vi "VI Linearisierung v2.vi"() -> ()   [LabVIEW 2020, in "Linearisierung v2.lvlib"]
uses:
  Linearisierung v2.lvlib
  Gasteiler/Stufen Tabelle.ctl
  Visualisierungs Elemente/Button.ctl
  Parameterkontrolle.ctl
  Visualisierungs Elemente/String - Eingabefeld.ctl
  SpanEinstellungen/SpanInletCluster.ctl
  Seiten/System Einstellungen V2/Konfig Gasflasche.ctl
  Seiten/System Einstellungen V2/Analysatoren.ctl
  Seiten/System Einstellungen V2/Gasflasche Auswahl.ctl
  SpanEinstellungen/Komponentencluster mit Formel.ctl
  SpanEinstellungen/Komponentenauswahl mit Formel.ctl
  SpanEinstellungen/Einheit.ctl
  Seiten/System Einstellungen V2/Traegergas.ctl
  Gasteiler/Gasteiler Stufen.ctl
  GasteilerType.ctl
  Visualisierungs Elemente/Zahlen-Ausgabefeld.ctl
  Gasteiler/Gasteiler Fehler.ctl
  Gasteiler/RS232.ctl
  Eingabetabelle.ctl
  Ausgabetabelle.ctl
  Auswahl Polynom Ordnung.ctl
  LIN Ausgabetabelle.ctl
  Visualisierungs Elemente/String - Ausgabefeld.ctl
  Gasnumber.ctl
  AktivArray.ctl
  AktivButton.ctl
  EPA Ausgabetabelle.ctl
  Visualisierungs Elemente/Pfad-Eingabefeld.ctl
  EPA Optionsfeld.ctl
  Gasteiler/HovaCal/Betriebsdaten.ctl
  Gasteiler/HovaCal/Gase.ctl
  Gasteiler/HovaCal/Vaporizer.ctl
  Gasteiler/HovaCal/Dynamsiche_Werte.ctl
  Polynomkoeffizientenanzeige.ctl
  Gasteiler/HovaCal/AutoLin Hovacal.ctl
  Seiten/CalGas Aufschaltung/Aufschaltung CalGas_ANZEIGE.ctl
  Visualisierungs Elemente/Auswahlfeld.ctl
  Kalibrieroption.ctl
  EPA1065-307/Condition.ctl
  Seiten/System Einstellungen V2/Gasteiler Auswahl.ctl
  Gasteiler/HovaCAL_Interface/Controls/Info Cluster Anzeige.ctl
  Gasteiler/HovaCAL_Interface/Controls/MFC Flow Anzeige.ctl
  Gasteiler/HovaCAL_Interface/Controls/Grenzen Anzeige.ctl
  Gasteiler/HovaCAL_Interface/Controls/Pumpe Modus Anzeige.ctl
  Gasteiler/HovaCAL_Interface/Controls/Pump Dry Mode Anzeige.ctl
  Gasteiler/HovaCAL_Interface/Controls/Pump Control Mode Anzeige.ctl
  Gasteiler/HovaCAL_Interface/Controls/Temp Ausgang Anzeige.ctl
  Gasteiler/HovaCAL_Interface/Controls/Temp Sollwerte Anzeige.ctl
  Gasteiler/HovaCAL_Interface/Controls/Flow Einstellung.ctl
  Gasteiler/HovaCAL_Interface/Controls/Flow Anzeige.ctl
  Gasteiler/HovaCAL_Interface/Controls/Pumpe Status Anzeige.ctl
  Gasteiler/HovaCAL_Interface/Controls/Pump state.ctl
  Gasteiler/HovaCAL_Interface/Controls/Pumpe MassenFluss Anzeige.ctl
  Gasteiler/HovaCAL_Interface/Controls/Pumpen Parameter Anzeige.ctl
  Gasteiler/HovaCAL_Interface/Controls/Reagent Anzeige.ctl
  Gasteiler/HovaCAL_Interface/Controls/Pump Concentration Mode Anzeige.ctl
  Gasteiler/HovaCAL_Interface/Controls/MFC Konfiguration.ctl
  Gasteiler/HovaCAL_Interface/Controls/MFC Einstellungen.ctl
  Gasteiler/HovaCAL_Interface/Controls/MFC Output.ctl
  Gasteiler/HovaCAL_Interface/Controls/Pumpen Output.ctl
  Visualisierungs Elemente/Checkbox(boolsch).ctl
  Seiten/CalGas Aufschaltung/Lin Modus.ctl
  Gasteiler/HovaCAL_Interface/Controls/Pumpen Parameter Anzeige Eingabe.ctl
  EPA 1065/T90 1065-308/Auswahl.ctl
  SpanEinstellungen/Aktion FGV Komponentenreferenz verwalten.ctl
  Seiten/FT-IR/FGV FT-IR Gasliste Aktionen.ctl
  Seiten/System Einstellungen V2/Aktion FGV Gasbottledefinition.ctl
  SpanEinstellungen/Aktion FGV SpanEinstellungen.ctl
  SpanEinstellungen/Aktion FGV Spans abarbeiten.ctl
  SpanEinstellungen/Aktion FGV SPAN Verriegelung.ctl
  Gasteiler/Aktion FGV Gasteilerliste laden.ctl
  SpanEinstellungen/Aktion FGV Post Processing.ctl
  SpanEinstellungen/Aktion FGV SPAN Stufentabellen.ctl
  Gasteiler/HovaCAL_Interface/Kommunikation/Aktion_FGV_HovaCAL_Interface_Kommandos.ctl
  Gasteiler/HovaCAL_Interface/Kommunikation/Aktion_FGV_HovaCAL_Interface_GetData.ctl
  Gasteiler/HovaCAL_Interface/Kommunikation/Aktion_FGV_HovaCAL_Interface_SetData.ctl
  Aktion Lin Daten aufarbeiten.ctl
  Gasteiler/Gasteiler Type.ctl
  Gasteiler/HovaCal/Aktion_FGV_Betriebsdaten.ctl
  LinV2 Registerkarten.ctl
  Seiten/CalGas Aufschaltung/FGV CalGas Aktionen.ctl
  Seiten/FT-IR/Span/Aktion FGV Span.ctl
  Gasteiler/Aktionen FGV Gasteiler Daten.ctl
  Aktion FGV Stoerungen sammeln und auswerten.ctl
  Aktion FGV Rohmesswerte sammeln.ctl
  Gasteiler/HovaCAL_Interface/Kommunikation/Aktion FGV HovaCAL Interface Autolin.ctl
  Aktionen Polynom Daten speichern.ctl
  Gasteiler/Aktion FGV Gasteiler Korrektur.ctl
  Gasteiler/Aktion FGV Daten Abholung uebergebenctl.ctl
  Gasteiler/HovaCAL_Interface/Kommunikation/Aktion_FGV_HovaCAL_Interface_Kommunikation.ctl
  Sprachverwaltung/FGV Aktion Tabelle zerlegen.ctl
  PDF_Interface/PDF Interface Helper/PDFResultPictures.ctl
  Seiten/FT-IR/Aktionen EVID-Codes.ctl
  EPA 1065/Allgemeine VIs/Aktion Wertaenderung Gasliste.ctl
  EPA 1065/Allgemeine VIs/Aktion Test Status.ctl
  Passwortverwaltung/FGV Passwort Aktion.ctl
  Gasteiler/AK-Komm Gasteiler/Aktionen AK Komm.ctl
  Gasteiler/AK-Komm Gasteiler/Alter Gasteiler/Aktionen AK Komm_ALT.ctl
  Gasteiler/Horiba/Aktion Befehl.ctl
  Gasteiler/HovaCAL_Interface/Kommunikation/Aktion_FGV_HovaCAL_Interface_Gasliste.ctl
  Seiten/System Einstellungen V2/Aktion FGV SystemEinstellungenV2.ctl
  Gasteiler/Gasteiler Daten.ctl
  Funktionstasten/Funktionstasten-Aktion.ctl
  Funktionstasten/Zustaende.ctl
  Auto Kalibrieren/Aktion FGV Autokal GT.ctl
  Seiten/EL3000/FID/FID Kalibrierung/FID Kalibrieren.ctl
  Seiten/EL3000/PMA/Kalibrieren/Kalibrierung O2.ctl
  Gasteiler/HovaCal/Aktion_FGV_Kom.ctl
  EPA1065-307/Aktion FGV Auswertung sammeln.ctl
  SpanEinstellungen/GD Abfrage Referenzen.ctl
  Aktion FGV GD Status Anzeige.ctl
  SpanEinstellungen/Aktion FGV GD Errors sammeln.ctl
  SpanEinstellungen/Postprocessing_Running_Indices.ctl
  LIN ErrorCluster.ctl
  Passwortverwaltung/Passwort.lvlib
  cRIO/PC/Kommunikation mit cRIO.lvlib
  Allgemein/allgemeine Sub-VIs.lvlib
  Seiten/FT-IR/FT-IR.lvlib
  Sprachverwaltung/Sprachverwaltung.lvlib
  Gasteiler/Gasteiler.lvlib
  Gasteiler/AK-Komm Gasteiler/Alter Gasteiler/Alter Gasteiler.lvlib
  Gasteiler/Horiba/Horiba GDC.lvlib
  Gasteiler/AK-Komm Gasteiler/AK Komm Gasteiler.lvlib
  Funktionstasten/Funktionstasten.lvlib
  EPA1065-307/Linearity verification 1065-307.lvlib
  Gasteiler/HovaCal/HovaCal.lvlib
  Seiten/EL3000/Allgemeine VI/Allgemeine VI.lvlib
  Seiten/EL3000/FID/FID Kalibrierung/FID Kalibrierung.lvlib
  Seiten/EL3000/PMA/Kalibrieren/Kalibrieren.lvlib
  Seiten/CalGas Aufschaltung/CalGas Aufschaltung.lvlib
  Seiten/FT-IR/Span/Spanfaktor.lvlib
  Auto Kalibrieren/Auto Kalibrieren.lvlib
  Seiten/FT-IR/TOOLweb Interface Library/TOOLweb Interface.lvlib
  Seiten/System Einstellungen V2/System Einstellungen V2.lvlib
  Gasteiler/HovaCAL_Interface/Kommunikation/Kommunikation.lvlib
  SpanEinstellungen/SpanEinstellungen.lvlib
  Protokoll/Protokoll.lvlib
  PDF_Interface/PDF Interface.lvlib
  <vilib>/Utility/miscctls.llb/LVRowAndColumnTypeDef.ctl
  Gasteiler/HovaCAL_Interface/Helper/Helper.lvlib
  EPA 1065/EPA 1065.lvlib
  PDF_Interface/PDF Interface Helper/PDF Interface Helper.lvlib
  EPA 1065/T90 1065-308/T90 Test 1065-308.lvlib
  Gasteiler/HovaCAL_Interface/HovaCAL_Interface.lvlib
  Gasteiler/HovaCAL_Interface/Controls/Controls.lvlib
panel:
  in  "Graphik für Messwerte":T1
  in  "EPA Optionsfeld":T2=enum."Rohwert"
  out "Ergebnis PDF FALSE":T3 caption="Ergebnis 2"
  out "Ergebnis PDF TRUE":T3 caption="Ergebnis 1"
  in  "Gasliste geändert":bool
  in  "Systemeinstellung":bool
  in  "Start LinCheck":T4
  in  "Kalibrierauswahl":T5 caption="Kalibrierung:" items=["Inaktiv", "Aktiv"]
  out "XY-Graph LIN 2":cluster{dbl[], dbl[]}[](graph) caption="XY-Graph"
  out "XY-Graph EPA 2":cluster{dbl[], dbl[]}[](graph) caption="XY-Graph"
  in  "Aufschaltung CalGas":T6 {"Aufschaltpunkt" items=["Filterblock", "Analysator direkt", "PNS", "Entnahme", "Gasdivider"]; "Kalibriergas" items=["Stickstoff"]}
  in  "Boolsch für LinStart":bool
  in  "Hauptregisterkarte":T8(tab)
  in  "Pfad Auto Lin":T9 caption="Pfad für Spans automatisch:"
  in  "PDF Deckblatt":T1 caption="Protokoll mit Deckblatt"
  in  "PDF single pages Components":T1 caption="Protokoll je Mischgas-Komponente separat erstellen"
  in  "PDF öffnen":T1 caption="Protokoll nach Linearisierung anzeigen"
  in  "use old LNI":T1
  in  "MG_use_magic_formula":T1=TRUE
  in  "Modus":T10 caption="Modus:" items=["Cal Gas zu PNS", "Cal Gas zu Entnahmestelle", "Messen"]
  in  "Gasteiler Span Eingänge":u16(ring)=128 caption="Span Eingänge nutzen:" items=["0", "1", "2", "3", "4", "5", "6", "7", "8", "9", "10"]
  in  "PDF single pages Span":T1 caption="Protokoll je Span separat erstellen"
  in  "automatisch":T1 caption="Span Einstellungen automatisieren"
  in  "Konfig Gasteiler":T11 caption="Gasteiler:" items=["----"=10000]
  in  "Lin laden":T4
  in  "Gasteilerkorrektur":T4
  in  "Bearbeiter":T12 caption="Bearbeiter:"
  in  "Registerkarte":enum32{"IP", "Serial"}(tab)
  in  "Serielle Parameter":T13={"VISA Resource Name"="COM1", "Baud Rate"=9600, "data bits"=8, "parity"=0, "stop bits"=10, "flow control"=0} {"stop bits" items=["1.0"=10, "1.5"=15, "2.0"=20]; "parity" items=["None", "Odd", "Even", "Mark", "Space"]; "flow control" items=["None"=0, "XON/XOFF"=1, "RTS/CTS"=2, "DTR/DSR"=4]; "data bits" items=["8"=8, "7"=7, "6"=6, "5"=5, "4"=4]; "Baud Rate" items=["115200"=115200, "38400"=38400, "19200"=19200, "14400"=14400, "9600"=9600, "4800"=4800, "2400"=2400]}
  in  "IP 4":u8
  in  "IP 3":u8
  in  "IP 2":u8
  in  "IP 1":u8
  in  "Port":u16 caption="Port:"
  in  "TCP Verbindung aktiv":bool
  out "Gasteilerstatus":string caption="Status:"
  out "Druck CG zu Gasteiler:":T14 caption="Druck CG:" format="%.1f"
  in  "Gasteiler Type":T15 items=["LNI", "Analog-Display", "AVL GDU", "Horiba GDC", "HovaCal", "Horiba SGD 710C"]
  in  "Gasteiler Stufen":T16=128 items=["10"=10, "11"=11, "16"=16, "32"=32, "64"=64, "128"=128, "256"=256, "500"=500, "1000"=1000]
  out "Störung Kommunikation":bool
  in  "Gasteiler":T12 caption="Gas Dividers"
  in  "Anforderung":T4
  out "Error":T17
  out "Störung Gasteiler":bool
  in  "Horiba GDC":T4 caption="Manuell"
  in  "SpanRegister":T18(tab)
  in  "Stufentabelle":enum32{"Span", "Punkte"}(tab)
  in  "Span 1":T19={"Span Inlet Active"=FALSE, "Analysator"="FT-IR", "Konfig Gasflasche"=FALSE, "Gasflasche"=0, "Gasflaschen Nr.:"="", "Ablaufdatum"=timestamp(0 s since 1904-01-01), "Komponenten"={"Komponente 1"={"Komponente:"=0, "Summenformel"="", "Konzentration IST"=0.0, "Einheit"=enum."ppm", "Genauigkeit"=0.0}, "Komponente 2"={"Komponente:"=0, "Summenformel"="", "Konzentration IST"=0.0, "Einheit"=enum."ppm", "Genauigkeit"=0.0}, "Komponente 3"={"Komponente:"=0, "Summenformel"="", "Konzentration IST"=0.0, "Einheit"=enum."ppm", "Genauigkeit"=0.0}, "Komponente 4"={"Komponente:"=0, "Summenformel"="", "Konzentration IST"=0.0, "Einheit"=enum."ppm", "Genauigkeit"=0.0}, "Komponente 5"={"Komponente:"=0, "Summenformel"="", "Konzentration IST"=0.0, "Einheit"=enum."ppm", "Genauigkeit"=0.0}}, "Zeitdauer Stufen"=0.0, "Max Fehler"=0.0, "Anzahl Stufen"=0.0, "Trägergas"="N2", "zusätzliche Zeitdauer Erster Punkt"=0.0} {"zusätzliche Zeitdauer Erster Punkt" min=30 step=1 format="%#_5g"; "Zeitdauer Stufen" format="%#_5g"; "Max Fehler" format="%#_5g"; "Anzahl Stufen" format="%#_5g"; "Komponenten"."Komponente 5"."Komponente:" items=["---"]; "Komponenten"."Komponente 5"."Konzentration IST" format="%#.4f"; "Komponenten"."Komponente 5"."Genauigkeit" format="%#.1f"; "Komponenten"."Komponente 4"."Komponente:" items=["---"]; "Komponenten"."Komponente 4"."Konzentration IST" format="%#.4f"; "Komponenten"."Komponente 4"."Genauigkeit" format="%#.1f"; "Komponenten"."Komponente 3"."Komponente:" items=["---"]; "Komponenten"."Komponente 3"."Konzentration IST" format="%#.4f"; "Komponenten"."Komponente 3"."Genauigkeit" format="%#.1f"; "Komponenten"."Komponente 2"."Komponente:" items=["---"]; "Komponenten"."Komponente 2"."Konzentration IST" format="%#.4f"; "Komponenten"."Komponente 2"."Genauigkeit" format="%#.1f"; "Komponenten"."Komponente 1"."Komponente:" items=["---"]; "Komponenten"."Komponente 1"."Konzentration IST" format="%#.4f"; "Komponenten"."Komponente 1"."Genauigkeit" format="%#.1f"; "Ablaufdatum" format="%<%d.%m.%Y>T"; "Gasflasche" items=["----"=10000]}
  in  "Stufen Tabelle":T27
  in  "Punkte umkehren":bool
  in  "Abfragen":T4
  out "Parameterkontrolle:":T28
  in  "PrüfgasName":T12 caption="Summenformel:"
  in  "auto Scan Points":bool
  in  "Stufentabelle 2":enum32{"Span", "Punkte"}(tab) caption="Stufentabelle"
  in  "Span 2":T19={"Span Inlet Active"=FALSE, "Analysator"="FT-IR", "Konfig Gasflasche"=FALSE, "Gasflasche"=0, "Gasflaschen Nr.:"="", "Ablaufdatum"=timestamp(0 s since 1904-01-01), "Komponenten"={"Komponente 1"={"Komponente:"=0, "Summenformel"="", "Konzentration IST"=0.0, "Einheit"=enum."ppm", "Genauigkeit"=0.0}, "Komponente 2"={"Komponente:"=0, "Summenformel"="", "Konzentration IST"=0.0, "Einheit"=enum."ppm", "Genauigkeit"=0.0}, "Komponente 3"={"Komponente:"=0, "Summenformel"="", "Konzentration IST"=0.0, "Einheit"=enum."ppm", "Genauigkeit"=0.0}, "Komponente 4"={"Komponente:"=0, "Summenformel"="", "Konzentration IST"=0.0, "Einheit"=enum."ppm", "Genauigkeit"=0.0}, "Komponente 5"={"Komponente:"=0, "Summenformel"="", "Konzentration IST"=0.0, "Einheit"=enum."ppm", "Genauigkeit"=0.0}}, "Zeitdauer Stufen"=0.0, "Max Fehler"=0.0, "Anzahl Stufen"=0.0, "Trägergas"="N2", "zusätzliche Zeitdauer Erster Punkt"=0.0} {"zusätzliche Zeitdauer Erster Punkt" min=30 step=1 format="%#_5g"; "Zeitdauer Stufen" format="%#_5g"; "Max Fehler" format="%#_5g"; "Anzahl Stufen" format="%#_5g"; "Komponenten"."Komponente 5"."Komponente:" items=["---"]; "Komponenten"."Komponente 5"."Konzentration IST" format="%#.4f"; "Komponenten"."Komponente 5"."Genauigkeit" format="%#.1f"; "Komponenten"."Komponente 4"."Komponente:" items=["---"]; "Komponenten"."Komponente 4"."Konzentration IST" format="%#.4f"; "Komponenten"."Komponente 4"."Genauigkeit" format="%#.1f"; "Komponenten"."Komponente 3"."Komponente:" items=["---"]; "Komponenten"."Komponente 3"."Konzentration IST" format="%#.4f"; "Komponenten"."Komponente 3"."Genauigkeit" format="%#.1f"; "Komponenten"."Komponente 2"."Komponente:" items=["---"]; "Komponenten"."Komponente 2"."Konzentration IST" format="%#.4f"; "Komponenten"."Komponente 2"."Genauigkeit" format="%#.1f"; "Komponenten"."Komponente 1"."Komponente:" items=["---"]; "Komponenten"."Komponente 1"."Konzentration IST" format="%#.4f"; "Komponenten"."Komponente 1"."Genauigkeit" format="%#.1f"; "Ablaufdatum" format="%<%d.%m.%Y>T"; "Gasflasche" items=["----"=10000]}
  in  "Stufen Tabelle 2":T27 caption="Stufen Tabelle"
  in  "Punkte umkehren 2":bool caption="Punkte umkehren"
  in  "Abfragen 2":T4 caption="Abfragen"
  out "Parameterkontrolle: 2":T28 caption="Parameterkontrolle:"
  in  "PrüfgasName 2":T12 caption="Summenformel:"
  in  "auto Scan Points 2":bool caption="auto Scan Points"
  in  "Stufentabelle 3":enum32{"Span", "Punkte"}(tab) caption="Stufentabelle"
  in  "Span 3":T19={"Span Inlet Active"=FALSE, "Analysator"="FT-IR", "Konfig Gasflasche"=FALSE, "Gasflasche"=0, "Gasflaschen Nr.:"="", "Ablaufdatum"=timestamp(0 s since 1904-01-01), "Komponenten"={"Komponente 1"={"Komponente:"=0, "Summenformel"="", "Konzentration IST"=0.0, "Einheit"=enum."ppm", "Genauigkeit"=0.0}, "Komponente 2"={"Komponente:"=0, "Summenformel"="", "Konzentration IST"=0.0, "Einheit"=enum."ppm", "Genauigkeit"=0.0}, "Komponente 3"={"Komponente:"=0, "Summenformel"="", "Konzentration IST"=0.0, "Einheit"=enum."ppm", "Genauigkeit"=0.0}, "Komponente 4"={"Komponente:"=0, "Summenformel"="", "Konzentration IST"=0.0, "Einheit"=enum."ppm", "Genauigkeit"=0.0}, "Komponente 5"={"Komponente:"=0, "Summenformel"="", "Konzentration IST"=0.0, "Einheit"=enum."ppm", "Genauigkeit"=0.0}}, "Zeitdauer Stufen"=0.0, "Max Fehler"=0.0, "Anzahl Stufen"=0.0, "Trägergas"="N2", "zusätzliche Zeitdauer Erster Punkt"=0.0} {"zusätzliche Zeitdauer Erster Punkt" min=30 step=1 format="%#_5g"; "Zeitdauer Stufen" format="%#_5g"; "Max Fehler" format="%#_5g"; "Anzahl Stufen" format="%#_5g"; "Komponenten"."Komponente 5"."Komponente:" items=["---"]; "Komponenten"."Komponente 5"."Konzentration IST" format="%#.4f"; "Komponenten"."Komponente 5"."Genauigkeit" format="%#.1f"; "Komponenten"."Komponente 4"."Komponente:" items=["---"]; "Komponenten"."Komponente 4"."Konzentration IST" format="%#.4f"; "Komponenten"."Komponente 4"."Genauigkeit" format="%#.1f"; "Komponenten"."Komponente 3"."Komponente:" items=["---"]; "Komponenten"."Komponente 3"."Konzentration IST" format="%#.4f"; "Komponenten"."Komponente 3"."Genauigkeit" format="%#.1f"; "Komponenten"."Komponente 2"."Komponente:" items=["---"]; "Komponenten"."Komponente 2"."Konzentration IST" format="%#.4f"; "Komponenten"."Komponente 2"."Genauigkeit" format="%#.1f"; "Komponenten"."Komponente 1"."Komponente:" items=["---"]; "Komponenten"."Komponente 1"."Konzentration IST" format="%#.4f"; "Komponenten"."Komponente 1"."Genauigkeit" format="%#.1f"; "Ablaufdatum" format="%<%d.%m.%Y>T"; "Gasflasche" items=["----"=10000]}
  in  "Stufen Tabelle 3":T27 caption="Stufen Tabelle"
  in  "Punkte umkehren 3":bool caption="Punkte umkehren"
  in  "Abfragen 3":T4 caption="Abfragen"
  out "Parameterkontrolle: 3":T28 caption="Parameterkontrolle:"
  in  "PrüfgasName 3":T12 caption="Summenformel:"
  in  "auto Scan Points 3":bool caption="auto Scan Points"
  in  "Stufentabelle 4":enum32{"Span", "Punkte"}(tab) caption="Stufentabelle"
  in  "Span 4":T19={"Span Inlet Active"=FALSE, "Analysator"="FT-IR", "Konfig Gasflasche"=FALSE, "Gasflasche"=0, "Gasflaschen Nr.:"="", "Ablaufdatum"=timestamp(0 s since 1904-01-01), "Komponenten"={"Komponente 1"={"Komponente:"=0, "Summenformel"="", "Konzentration IST"=0.0, "Einheit"=enum."ppm", "Genauigkeit"=0.0}, "Komponente 2"={"Komponente:"=0, "Summenformel"="", "Konzentration IST"=0.0, "Einheit"=enum."ppm", "Genauigkeit"=0.0}, "Komponente 3"={"Komponente:"=0, "Summenformel"="", "Konzentration IST"=0.0, "Einheit"=enum."ppm", "Genauigkeit"=0.0}, "Komponente 4"={"Komponente:"=0, "Summenformel"="", "Konzentration IST"=0.0, "Einheit"=enum."ppm", "Genauigkeit"=0.0}, "Komponente 5"={"Komponente:"=0, "Summenformel"="", "Konzentration IST"=0.0, "Einheit"=enum."ppm", "Genauigkeit"=0.0}}, "Zeitdauer Stufen"=0.0, "Max Fehler"=0.0, "Anzahl Stufen"=0.0, "Trägergas"="N2", "zusätzliche Zeitdauer Erster Punkt"=0.0} {"zusätzliche Zeitdauer Erster Punkt" min=30 step=1 format="%#_5g"; "Zeitdauer Stufen" format="%#_5g"; "Max Fehler" format="%#_5g"; "Anzahl Stufen" format="%#_5g"; "Komponenten"."Komponente 5"."Komponente:" items=["---"]; "Komponenten"."Komponente 5"."Konzentration IST" format="%#.4f"; "Komponenten"."Komponente 5"."Genauigkeit" format="%#.1f"; "Komponenten"."Komponente 4"."Komponente:" items=["---"]; "Komponenten"."Komponente 4"."Konzentration IST" format="%#.4f"; "Komponenten"."Komponente 4"."Genauigkeit" format="%#.1f"; "Komponenten"."Komponente 3"."Komponente:" items=["---"]; "Komponenten"."Komponente 3"."Konzentration IST" format="%#.4f"; "Komponenten"."Komponente 3"."Genauigkeit" format="%#.1f"; "Komponenten"."Komponente 2"."Komponente:" items=["---"]; "Komponenten"."Komponente 2"."Konzentration IST" format="%#.4f"; "Komponenten"."Komponente 2"."Genauigkeit" format="%#.1f"; "Komponenten"."Komponente 1"."Komponente:" items=["---"]; "Komponenten"."Komponente 1"."Konzentration IST" format="%#.4f"; "Komponenten"."Komponente 1"."Genauigkeit" format="%#.1f"; "Ablaufdatum" format="%<%d.%m.%Y>T"; "Gasflasche" items=["----"=10000]}
  in  "Stufen Tabelle 4":T27 caption="Stufen Tabelle"
  in  "Punkte umkehren 4":bool caption="Punkte umkehren"
  in  "Abfragen 4":T4 caption="Abfragen"
  out "Parameterkontrolle: 4":T28 caption="Parameterkontrolle:"
  in  "PrüfgasName 4":T12 caption="Summenformel:"
  in  "auto Scan Points 4":bool caption="auto Scan Points"
  in  "Stufentabelle 5":enum32{"Span", "Punkte"}(tab) caption="Stufentabelle"
  in  "Span 5":T19={"Span Inlet Active"=FALSE, "Analysator"="FT-IR", "Konfig Gasflasche"=FALSE, "Gasflasche"=0, "Gasflaschen Nr.:"="", "Ablaufdatum"=timestamp(0 s since 1904-01-01), "Komponenten"={"Komponente 1"={"Komponente:"=0, "Summenformel"="", "Konzentration IST"=0.0, "Einheit"=enum."ppm", "Genauigkeit"=0.0}, "Komponente 2"={"Komponente:"=0, "Summenformel"="", "Konzentration IST"=0.0, "Einheit"=enum."ppm", "Genauigkeit"=0.0}, "Komponente 3"={"Komponente:"=0, "Summenformel"="", "Konzentration IST"=0.0, "Einheit"=enum."ppm", "Genauigkeit"=0.0}, "Komponente 4"={"Komponente:"=0, "Summenformel"="", "Konzentration IST"=0.0, "Einheit"=enum."ppm", "Genauigkeit"=0.0}, "Komponente 5"={"Komponente:"=0, "Summenformel"="", "Konzentration IST"=0.0, "Einheit"=enum."ppm", "Genauigkeit"=0.0}}, "Zeitdauer Stufen"=0.0, "Max Fehler"=0.0, "Anzahl Stufen"=0.0, "Trägergas"="N2", "zusätzliche Zeitdauer Erster Punkt"=0.0} {"zusätzliche Zeitdauer Erster Punkt" min=30 step=1 format="%#_5g"; "Zeitdauer Stufen" format="%#_5g"; "Max Fehler" format="%#_5g"; "Anzahl Stufen" format="%#_5g"; "Komponenten"."Komponente 5"."Komponente:" items=["---"]; "Komponenten"."Komponente 5"."Konzentration IST" format="%#.4f"; "Komponenten"."Komponente 5"."Genauigkeit" format="%#.1f"; "Komponenten"."Komponente 4"."Komponente:" items=["---"]; "Komponenten"."Komponente 4"."Konzentration IST" format="%#.4f"; "Komponenten"."Komponente 4"."Genauigkeit" format="%#.1f"; "Komponenten"."Komponente 3"."Komponente:" items=["---"]; "Komponenten"."Komponente 3"."Konzentration IST" format="%#.4f"; "Komponenten"."Komponente 3"."Genauigkeit" format="%#.1f"; "Komponenten"."Komponente 2"."Komponente:" items=["---"]; "Komponenten"."Komponente 2"."Konzentration IST" format="%#.4f"; "Komponenten"."Komponente 2"."Genauigkeit" format="%#.1f"; "Komponenten"."Komponente 1"."Komponente:" items=["---"]; "Komponenten"."Komponente 1"."Konzentration IST" format="%#.4f"; "Komponenten"."Komponente 1"."Genauigkeit" format="%#.1f"; "Ablaufdatum" format="%<%d.%m.%Y>T"; "Gasflasche" items=["----"=10000]}
  in  "Stufen Tabelle 5":T27 caption="Stufen Tabelle"
  in  "Punkte umkehren 5":bool caption="Punkte umkehren"
  in  "Abfragen 5":T4 caption="Abfragen"
  out "Parameterkontrolle: 5":T28 caption="Parameterkontrolle:"
  in  "PrüfgasName 5":T12 caption="Summenformel:"
  in  "auto Scan Points 5":bool caption="auto Scan Points"
  in  "Stufentabelle 6":enum32{"Span", "Punkte"}(tab) caption="Stufentabelle"
  in  "Span 6":T19={"Span Inlet Active"=FALSE, "Analysator"="FT-IR", "Konfig Gasflasche"=FALSE, "Gasflasche"=0, "Gasflaschen Nr.:"="", "Ablaufdatum"=timestamp(0 s since 1904-01-01), "Komponenten"={"Komponente 1"={"Komponente:"=0, "Summenformel"="", "Konzentration IST"=0.0, "Einheit"=enum."ppm", "Genauigkeit"=0.0}, "Komponente 2"={"Komponente:"=0, "Summenformel"="", "Konzentration IST"=0.0, "Einheit"=enum."ppm", "Genauigkeit"=0.0}, "Komponente 3"={"Komponente:"=0, "Summenformel"="", "Konzentration IST"=0.0, "Einheit"=enum."ppm", "Genauigkeit"=0.0}, "Komponente 4"={"Komponente:"=0, "Summenformel"="", "Konzentration IST"=0.0, "Einheit"=enum."ppm", "Genauigkeit"=0.0}, "Komponente 5"={"Komponente:"=0, "Summenformel"="", "Konzentration IST"=0.0, "Einheit"=enum."ppm", "Genauigkeit"=0.0}}, "Zeitdauer Stufen"=0.0, "Max Fehler"=0.0, "Anzahl Stufen"=0.0, "Trägergas"="N2", "zusätzliche Zeitdauer Erster Punkt"=0.0} {"zusätzliche Zeitdauer Erster Punkt" min=30 step=1 format="%#_5g"; "Zeitdauer Stufen" format="%#_5g"; "Max Fehler" format="%#_5g"; "Anzahl Stufen" format="%#_5g"; "Komponenten"."Komponente 5"."Komponente:" items=["---"]; "Komponenten"."Komponente 5"."Konzentration IST" format="%#.4f"; "Komponenten"."Komponente 5"."Genauigkeit" format="%#.1f"; "Komponenten"."Komponente 4"."Komponente:" items=["---"]; "Komponenten"."Komponente 4"."Konzentration IST" format="%#.4f"; "Komponenten"."Komponente 4"."Genauigkeit" format="%#.1f"; "Komponenten"."Komponente 3"."Komponente:" items=["---"]; "Komponenten"."Komponente 3"."Konzentration IST" format="%#.4f"; "Komponenten"."Komponente 3"."Genauigkeit" format="%#.1f"; "Komponenten"."Komponente 2"."Komponente:" items=["---"]; "Komponenten"."Komponente 2"."Konzentration IST" format="%#.4f"; "Komponenten"."Komponente 2"."Genauigkeit" format="%#.1f"; "Komponenten"."Komponente 1"."Komponente:" items=["---"]; "Komponenten"."Komponente 1"."Konzentration IST" format="%#.4f"; "Komponenten"."Komponente 1"."Genauigkeit" format="%#.1f"; "Ablaufdatum" format="%<%d.%m.%Y>T"; "Gasflasche" items=["----"=10000]}
  in  "Stufen Tabelle 6":T27 caption="Stufen Tabelle"
  in  "Punkte umkehren 6":bool caption="Punkte umkehren"
  in  "Abfragen 6":T4 caption="Abfragen"
  out "Parameterkontrolle: 6":T28 caption="Parameterkontrolle:"
  in  "PrüfgasName 6":T12 caption="Summenformel:"
  in  "auto Scan Points 6":bool caption="auto Scan Points"
  in  "Stufentabelle 7":enum32{"Span", "Punkte"}(tab) caption="Stufentabelle"
  in  "Span 7":T19={"Span Inlet Active"=FALSE, "Analysator"="FT-IR", "Konfig Gasflasche"=FALSE, "Gasflasche"=0, "Gasflaschen Nr.:"="", "Ablaufdatum"=timestamp(0 s since 1904-01-01), "Komponenten"={"Komponente 1"={"Komponente:"=0, "Summenformel"="", "Konzentration IST"=0.0, "Einheit"=enum."ppm", "Genauigkeit"=0.0}, "Komponente 2"={"Komponente:"=0, "Summenformel"="", "Konzentration IST"=0.0, "Einheit"=enum."ppm", "Genauigkeit"=0.0}, "Komponente 3"={"Komponente:"=0, "Summenformel"="", "Konzentration IST"=0.0, "Einheit"=enum."ppm", "Genauigkeit"=0.0}, "Komponente 4"={"Komponente:"=0, "Summenformel"="", "Konzentration IST"=0.0, "Einheit"=enum."ppm", "Genauigkeit"=0.0}, "Komponente 5"={"Komponente:"=0, "Summenformel"="", "Konzentration IST"=0.0, "Einheit"=enum."ppm", "Genauigkeit"=0.0}}, "Zeitdauer Stufen"=0.0, "Max Fehler"=0.0, "Anzahl Stufen"=0.0, "Trägergas"="N2", "zusätzliche Zeitdauer Erster Punkt"=0.0} {"zusätzliche Zeitdauer Erster Punkt" min=30 step=1 format="%#_5g"; "Zeitdauer Stufen" format="%#_5g"; "Max Fehler" format="%#_5g"; "Anzahl Stufen" format="%#_5g"; "Komponenten"."Komponente 5"."Komponente:" items=["---"]; "Komponenten"."Komponente 5"."Konzentration IST" format="%#.4f"; "Komponenten"."Komponente 5"."Genauigkeit" format="%#.1f"; "Komponenten"."Komponente 4"."Komponente:" items=["---"]; "Komponenten"."Komponente 4"."Konzentration IST" format="%#.4f"; "Komponenten"."Komponente 4"."Genauigkeit" format="%#.1f"; "Komponenten"."Komponente 3"."Komponente:" items=["---"]; "Komponenten"."Komponente 3"."Konzentration IST" format="%#.4f"; "Komponenten"."Komponente 3"."Genauigkeit" format="%#.1f"; "Komponenten"."Komponente 2"."Komponente:" items=["---"]; "Komponenten"."Komponente 2"."Konzentration IST" format="%#.4f"; "Komponenten"."Komponente 2"."Genauigkeit" format="%#.1f"; "Komponenten"."Komponente 1"."Komponente:" items=["---"]; "Komponenten"."Komponente 1"."Konzentration IST" format="%#.4f"; "Komponenten"."Komponente 1"."Genauigkeit" format="%#.1f"; "Ablaufdatum" format="%<%d.%m.%Y>T"; "Gasflasche" items=["----"=10000]}
  in  "Stufen Tabelle 7":T27 caption="Stufen Tabelle"
  in  "Punkte umkehren 7":bool caption="Punkte umkehren"
  in  "Abfragen 7":T4 caption="Abfragen"
  out "Parameterkontrolle: 7":T28 caption="Parameterkontrolle:"
  in  "PrüfgasName 7":T12 caption="Summenformel:"
  in  "auto Scan Points 7":bool caption="auto Scan Points"
  in  "Stufentabelle 8":enum32{"Span", "Punkte"}(tab) caption="Stufentabelle"
  in  "Span 8":T19={"Span Inlet Active"=FALSE, "Analysator"="FT-IR", "Konfig Gasflasche"=FALSE, "Gasflasche"=0, "Gasflaschen Nr.:"="", "Ablaufdatum"=timestamp(0 s since 1904-01-01), "Komponenten"={"Komponente 1"={"Komponente:"=0, "Summenformel"="", "Konzentration IST"=0.0, "Einheit"=enum."ppm", "Genauigkeit"=0.0}, "Komponente 2"={"Komponente:"=0, "Summenformel"="", "Konzentration IST"=0.0, "Einheit"=enum."ppm", "Genauigkeit"=0.0}, "Komponente 3"={"Komponente:"=0, "Summenformel"="", "Konzentration IST"=0.0, "Einheit"=enum."ppm", "Genauigkeit"=0.0}, "Komponente 4"={"Komponente:"=0, "Summenformel"="", "Konzentration IST"=0.0, "Einheit"=enum."ppm", "Genauigkeit"=0.0}, "Komponente 5"={"Komponente:"=0, "Summenformel"="", "Konzentration IST"=0.0, "Einheit"=enum."ppm", "Genauigkeit"=0.0}}, "Zeitdauer Stufen"=0.0, "Max Fehler"=0.0, "Anzahl Stufen"=0.0, "Trägergas"="N2", "zusätzliche Zeitdauer Erster Punkt"=0.0} {"zusätzliche Zeitdauer Erster Punkt" min=30 step=1 format="%#_5g"; "Zeitdauer Stufen" format="%#_5g"; "Max Fehler" format="%#_5g"; "Anzahl Stufen" format="%#_5g"; "Komponenten"."Komponente 5"."Komponente:" items=["---"]; "Komponenten"."Komponente 5"."Konzentration IST" format="%#.4f"; "Komponenten"."Komponente 5"."Genauigkeit" format="%#.1f"; "Komponenten"."Komponente 4"."Komponente:" items=["---"]; "Komponenten"."Komponente 4"."Konzentration IST" format="%#.4f"; "Komponenten"."Komponente 4"."Genauigkeit" format="%#.1f"; "Komponenten"."Komponente 3"."Komponente:" items=["---"]; "Komponenten"."Komponente 3"."Konzentration IST" format="%#.4f"; "Komponenten"."Komponente 3"."Genauigkeit" format="%#.1f"; "Komponenten"."Komponente 2"."Komponente:" items=["---"]; "Komponenten"."Komponente 2"."Konzentration IST" format="%#.4f"; "Komponenten"."Komponente 2"."Genauigkeit" format="%#.1f"; "Komponenten"."Komponente 1"."Komponente:" items=["---"]; "Komponenten"."Komponente 1"."Konzentration IST" format="%#.4f"; "Komponenten"."Komponente 1"."Genauigkeit" format="%#.1f"; "Ablaufdatum" format="%<%d.%m.%Y>T"; "Gasflasche" items=["----"=10000]}
  in  "Stufen Tabelle 8":T27 caption="Stufen Tabelle"
  in  "Punkte umkehren 8":bool caption="Punkte umkehren"
  in  "Abfragen 8":T4 caption="Abfragen"
  out "Parameterkontrolle: 8":T28 caption="Parameterkontrolle:"
  in  "PrüfgasName 8":T12 caption="Summenformel:"
  in  "auto Scan Points 8":bool caption="auto Scan Points"
  in  "Stufentabelle 9":enum32{"Span", "Punkte"}(tab) caption="Stufentabelle"
  in  "Span 9":T19={"Span Inlet Active"=FALSE, "Analysator"="FT-IR", "Konfig Gasflasche"=FALSE, "Gasflasche"=0, "Gasflaschen Nr.:"="", "Ablaufdatum"=timestamp(0 s since 1904-01-01), "Komponenten"={"Komponente 1"={"Komponente:"=0, "Summenformel"="", "Konzentration IST"=0.0, "Einheit"=enum."ppm", "Genauigkeit"=0.0}, "Komponente 2"={"Komponente:"=0, "Summenformel"="", "Konzentration IST"=0.0, "Einheit"=enum."ppm", "Genauigkeit"=0.0}, "Komponente 3"={"Komponente:"=0, "Summenformel"="", "Konzentration IST"=0.0, "Einheit"=enum."ppm", "Genauigkeit"=0.0}, "Komponente 4"={"Komponente:"=0, "Summenformel"="", "Konzentration IST"=0.0, "Einheit"=enum."ppm", "Genauigkeit"=0.0}, "Komponente 5"={"Komponente:"=0, "Summenformel"="", "Konzentration IST"=0.0, "Einheit"=enum."ppm", "Genauigkeit"=0.0}}, "Zeitdauer Stufen"=0.0, "Max Fehler"=0.0, "Anzahl Stufen"=0.0, "Trägergas"="N2", "zusätzliche Zeitdauer Erster Punkt"=0.0} {"zusätzliche Zeitdauer Erster Punkt" min=30 step=1 format="%#_5g"; "Zeitdauer Stufen" format="%#_5g"; "Max Fehler" format="%#_5g"; "Anzahl Stufen" format="%#_5g"; "Komponenten"."Komponente 5"."Komponente:" items=["---"]; "Komponenten"."Komponente 5"."Konzentration IST" format="%#.4f"; "Komponenten"."Komponente 5"."Genauigkeit" format="%#.1f"; "Komponenten"."Komponente 4"."Komponente:" items=["---"]; "Komponenten"."Komponente 4"."Konzentration IST" format="%#.4f"; "Komponenten"."Komponente 4"."Genauigkeit" format="%#.1f"; "Komponenten"."Komponente 3"."Komponente:" items=["---"]; "Komponenten"."Komponente 3"."Konzentration IST" format="%#.4f"; "Komponenten"."Komponente 3"."Genauigkeit" format="%#.1f"; "Komponenten"."Komponente 2"."Komponente:" items=["---"]; "Komponenten"."Komponente 2"."Konzentration IST" format="%#.4f"; "Komponenten"."Komponente 2"."Genauigkeit" format="%#.1f"; "Komponenten"."Komponente 1"."Komponente:" items=["---"]; "Komponenten"."Komponente 1"."Konzentration IST" format="%#.4f"; "Komponenten"."Komponente 1"."Genauigkeit" format="%#.1f"; "Ablaufdatum" format="%<%d.%m.%Y>T"; "Gasflasche" items=["----"=10000]}
  in  "Stufen Tabelle 9":T27 caption="Stufen Tabelle"
  in  "Punkte umkehren 9":bool caption="Punkte umkehren"
  in  "Abfragen 9":T4 caption="Abfragen"
  out "Parameterkontrolle: 9":T28 caption="Parameterkontrolle:"
  in  "PrüfgasName 9":T12 caption="Summenformel:"
  in  "auto Scan Points 9":bool caption="auto Scan Points"
  in  "Stufentabelle 10":enum32{"Span", "Punkte"}(tab) caption="Stufentabelle"
  in  "Span 10":T19={"Span Inlet Active"=FALSE, "Analysator"="FT-IR", "Konfig Gasflasche"=FALSE, "Gasflasche"=0, "Gasflaschen Nr.:"="", "Ablaufdatum"=timestamp(0 s since 1904-01-01), "Komponenten"={"Komponente 1"={"Komponente:"=0, "Summenformel"="", "Konzentration IST"=0.0, "Einheit"=enum."ppm", "Genauigkeit"=0.0}, "Komponente 2"={"Komponente:"=0, "Summenformel"="", "Konzentration IST"=0.0, "Einheit"=enum."ppm", "Genauigkeit"=0.0}, "Komponente 3"={"Komponente:"=0, "Summenformel"="", "Konzentration IST"=0.0, "Einheit"=enum."ppm", "Genauigkeit"=0.0}, "Komponente 4"={"Komponente:"=0, "Summenformel"="", "Konzentration IST"=0.0, "Einheit"=enum."ppm", "Genauigkeit"=0.0}, "Komponente 5"={"Komponente:"=0, "Summenformel"="", "Konzentration IST"=0.0, "Einheit"=enum."ppm", "Genauigkeit"=0.0}}, "Zeitdauer Stufen"=0.0, "Max Fehler"=0.0, "Anzahl Stufen"=0.0, "Trägergas"="N2", "zusätzliche Zeitdauer Erster Punkt"=0.0} {"zusätzliche Zeitdauer Erster Punkt" min=30 step=1 format="%#_5g"; "Zeitdauer Stufen" format="%#_5g"; "Max Fehler" format="%#_5g"; "Anzahl Stufen" format="%#_5g"; "Komponenten"."Komponente 5"."Komponente:" items=["---"]; "Komponenten"."Komponente 5"."Konzentration IST" format="%#.4f"; "Komponenten"."Komponente 5"."Genauigkeit" format="%#.1f"; "Komponenten"."Komponente 4"."Komponente:" items=["---"]; "Komponenten"."Komponente 4"."Konzentration IST" format="%#.4f"; "Komponenten"."Komponente 4"."Genauigkeit" format="%#.1f"; "Komponenten"."Komponente 3"."Komponente:" items=["---"]; "Komponenten"."Komponente 3"."Konzentration IST" format="%#.4f"; "Komponenten"."Komponente 3"."Genauigkeit" format="%#.1f"; "Komponenten"."Komponente 2"."Komponente:" items=["---"]; "Komponenten"."Komponente 2"."Konzentration IST" format="%#.4f"; "Komponenten"."Komponente 2"."Genauigkeit" format="%#.1f"; "Komponenten"."Komponente 1"."Komponente:" items=["---"]; "Komponenten"."Komponente 1"."Konzentration IST" format="%#.4f"; "Komponenten"."Komponente 1"."Genauigkeit" format="%#.1f"; "Ablaufdatum" format="%<%d.%m.%Y>T"; "Gasflasche" items=["----"=10000]}
  in  "Stufen Tabelle 10":T27 caption="Stufen Tabelle"
  in  "Punkte umkehren 10":bool caption="Punkte umkehren"
  in  "Abfragen 10":T4 caption="Abfragen"
  out "Parameterkontrolle: 10":T28 caption="Parameterkontrolle:"
  in  "PrüfgasName 10":T12 caption="Summenformel:"
  in  "auto Scan Points 10":bool caption="auto Scan Points"
  in  "HovaCALInterface-Freigabe":T4
  in  "HovaCALInterfaceInternal":enum32{"Configuration", "Data", "Info"}(tab)
  out "HovaCAL SetPumpMode-Cluster out":T29 caption="Pumpe Parameter" {"concentratio mode" items=["water", "reagent"]; "Reagent" items=["HCl", "HF", "NH3", "HG", "PPM", "ORGANIC"]}
  in  "Pump state for LIN":T32 caption="Pump start for LIN"
  in  "HovaCAL SetPumpMode":T32 caption="Pumpe manuell"
  in  "HovaCAL Flow AutoLin":T33 caption="Flow Setpoint LIN" {"HovaCAL Flow Input Cluster" format="%.2f"}
  in  "HovaCAL Flow Input Cluster":T33 caption="Fluss Sollwert manuell" {"HovaCAL Flow Input Cluster" format="%.2f"}
  out "Cluster.Flow Output Cluster (Ausgang)":T34 caption="Fluss Ausgang" {"Actual Flow" format="%.2f"}
  in  "HovaCAL SetPumpMode-Cluster":T35 caption="Pumpe Parameter" {"concentratio mode" items=["water", "reagent"]; "Reagent" items=["HCl", "HF", "NH3", "HG", "PPM", "ORGANIC"]}
  in  "HovaCAL Cluster.PumpModeGeneral":T36 caption="Pumpe Modus" {"dry mode" items=["wet", "dry"]; "control mode" items=["static", "pid"]}
  out "Cluster.PumpModeGeneral-Cluster":T39 caption="Pump Status"
  out "Cluster.Pump MassFlow-Cluster":T40 caption="Pumpe MassenFluss"
  in  "HovaCAL Limits Cluster":T41 caption="Grenzen"
  in  "HovaCAL Temperature":T42 caption="Temp Sollwerte" format="%.2f"
  out "Cluster.Temp Cluster":T43 caption="Temp Ausgang"
  out "Cluster.PumpModeGeneral-Cluster 2":T39 caption="Pump Status"
  out "Cluster.Flow Output Cluster (Ausgang) 2":T34 caption="Fluss Ausgang" {"Actual Flow" format="%.2f"}
  in  "MFC4":T44 caption="MFC5" {"Output Setpoint" format="%.2f"; "Input Concentration" format="%.2f"}
  in  "fix+MFC5":bool
  in  "fix+MFC4":bool
  in  "fix+MFC3":bool
  in  "fix+MFC2":bool
  in  "fix+MFC1":bool
  in  "HovaCAL MFC5 Komponente:":u16(ring) caption="Komponente:" items=["---"]
  in  "HovaCAL MFC4 Komponente:":u16(ring) caption="Komponente:" items=["---"]
  in  "HovaCAL MFC3 Komponente:":u16(ring) caption="Komponente:" items=["---"]
  in  "HovaCAL MFC2 Komponente:":u16(ring) caption="Komponente:" items=["---"]
  in  "HovaCAL MFC1 Komponente:":u16(ring) caption="Komponente:" items=["---"]
  out "MFC Output 2":T45 {"flow expected" format="%.2f"; "flow actual" format="%.2f"; "output concentration dry" format="%.2f"; "output concentration" format="%.2f"}
  in  "MFC0":T44 caption="MFC1" {"Output Setpoint" format="%.2f"; "Input Concentration" format="%.2f"}
  in  "MFC1":T44 caption="MFC2" {"Output Setpoint" format="%.2f"; "Input Concentration" format="%.2f"}
  in  "MFC2":T44 caption="MFC3" {"Output Setpoint" format="%.2f"; "Input Concentration" format="%.2f"}
  out "MFC Output 0":T45 {"flow expected" format="%.2f"; "flow actual" format="%.2f"; "output concentration dry" format="%.2f"; "output concentration" format="%.2f"}
  out "MFC Output 1":T45 {"flow expected" format="%.2f"; "flow actual" format="%.2f"; "output concentration dry" format="%.2f"; "output concentration" format="%.2f"}
  in  "HovaCAL MFC Gase Cluster 3":T46 caption="MFC Gase" {"MFC Gasauswahl" items=["AIR"]}
  in  "HovaCAL MFC Gase Cluster 2":T46 caption="MFC Gase" {"MFC Gasauswahl" items=["AIR", "O2-20%", "C3H8%2", "NO5000", "MG", "CO2-15%"]}
  in  "HovaCAL MFC Gase Cluster 1":T46 caption="MFC Gase" {"MFC Gasauswahl" items=["AIR"]}
  out "MFC Output 4":T45 {"flow expected" format="%.2f"; "flow actual" format="%.2f"; "output concentration dry" format="%.2f"; "output concentration" format="%.2f"}
  out "MFC Output 3":T45 {"flow expected" format="%.2f"; "flow actual" format="%.2f"; "output concentration dry" format="%.2f"; "output concentration" format="%.2f"}
  in  "MFC3":T44 caption="MFC4" {"Output Setpoint" format="%.2f"; "Input Concentration" format="%.2f"}
  in  "HovaCAL MFC Gase Cluster 5":T46 caption="MFC Gase" {"MFC Gasauswahl" items=["AIR"]}
  in  "HovaCAL MFC Gase Cluster 4":T46 caption="MFC Gase" {"MFC Gasauswahl" items=["AIR"]}
  in  "fix+Pump2":bool
  in  "fix+Pump1":bool
  in  "HovaCAL Pump2 Komponente:":u16(ring) caption="Komponente:" items=["---"]
  in  "HovaCAL Pump1 Komponente:":u16(ring) caption="Komponente:" items=["---"]
  out "Pump Output 2":T47 {"speed" format="%.2f"; "water conc dry" format="%.2f"; "water conc" format="%.2f"; "reagent conc dry" format="%.2f"; "reagent conc" format="%.2f"}
  out "Pump Output 1":T47 {"speed" format="%.2f"; "water conc dry" format="%.2f"; "water conc" format="%.2f"; "reagent conc dry" format="%.2f"; "reagent conc" format="%.2f"}
  in  "Pump 2":T44 caption="Pumpe/Spritzen 2" {"Output Setpoint" format="%.2f"; "Input Concentration" format="%.2f"}
  in  "Pump 1":T44 caption="Pumpe/Spritzen 1" {"Output Setpoint" format="%.2f"; "Input Concentration" format="%.2f"}
  in  "HovaCAL AutoLin MFC":u16(ring) caption="MFC/Pumpe Auswahl für Lin" items=["MFC1", "MFC2", "MFC3", "Pump0"]
  out "Komponente HovaCal Interface":T48 caption="Komponente"
  in  "Gasnummer HovaCal Interface":T49=1 caption="Komponente:" min=1 max=5
  out "Error 2":T17 caption="Error"
  out "Störung Kommunikation 2":bool caption="Störung Kommunikation"
  out "System Cluster":T50 caption="System Information"
  out "MFC Flow Cluster":T51 caption="MFC Flow"
  in  "PMD  E kalibrieren":T4 caption="PMD kalibrieren"
  in  "PMD 0 kalibrieren":T4 caption="PMD kalibrieren"
  in  "Gasteiler EP spülen":T4
  out "Status kalibrieren":string caption="Status"
  in  "FTIR Kalibrieren":T4 caption="Lin laden"
  in  "Gasteiler Spülen":T4
  in  "Kalibrier Optionen:":enum32{"Gasteiler", "ohne Gasteiler", "PNS"}(radio)
  in  "PMD kalibrieren":T4
  in  "FID 0 kalibrieren":T4 caption="FID kalibrieren"
  in  "FID E kalibrieren":T4 caption="FID kalibrieren"
  in  "FID kalibrieren":T4
  in  "post processing PDFs":T4
  in  "post processing done":T4 caption="DONE"
  in  "post processing":u16(ring) caption="Nachbearbeitung:" items=["---"]
  in  "passive Komponente:":u16(ring) items=["---"]
  out "Restlaufzeit":T14 caption="Restlaufzeit:"
  out "Einheit":string
  out "Istwert":T14 caption="Istwert:" format="%.2f"
  out "Schwankung":T14 caption="Standardabweichung:" format="%.2f"
  out "Einheit Deviation":string caption="Einheit"
  in  "FORTSETZEN":T4 caption="START"
  out "Polynom":T52 caption="Polynomkoeffizient:" {"O. 4" format="%#.18f"; "O. 3" format="%#.18f"; "O. 2" format="%#.18f"; "O.1" format="%#.18f"; "Offset" format="%#.18f"}
  in  "Istwerte löschen":T4 caption="Istwerte Abholen"
  in  "Alles löschen":T4 caption="Istwerte Abholen"
  out "Status":string
  out "Komponente Daten Gen":T48 caption="Komponente"
  in  "Gasnummer Generieren":T49=1 caption="Komponente:" min=1 max=5
  out "Ausgabetabelle":T53
  in  "Eingabetabelle":T54
  in  "Istwerte Abholen":T4
  in  "STARTEN":T4 caption="START"
  in  "ABBRECHEN":T4
  out "Offset":string caption="Offset:"
  out "Spanfactor":string caption="Spanfaktor:"
  in  "LIN Filename override":T1 caption="eigener Dateiname und Pfad verwenden"
  out "LIN Polynomkoeffizienten":T52 caption="Polynomkoeffizient:" {"O. 4" format="%#.18f"; "O. 3" format="%#.18f"; "O. 2" format="%#.18f"; "O.1" format="%#.18f"; "Offset" format="%#.18f"}
  out "LIN Max. Error in %:":sgl caption="Max. Error in %:" format="%#.2f"
  in  "Polynom-Ordnung":T55
  in  "Neue Polynom":T4
  out "Komponentenanzeige LIN":T48 caption="Komponente"
  in  "Gasnummer LIN":T49=1 caption="Komponente:" min=1 max=5
  out "LIN Ausgabetabelle":T56
  in  "Aktiv LIN":T57
  out "XY-Graph LIN":cluster{dbl[], dbl[]}[](graph) caption="XY-Graph"
  in  "Pfad LIN":T9 caption="Pfad"
  in  "Speichern LIN":T4 caption="SPEICHERN"
  in  "File Name LIN":T12 caption="File Name"
  out "Spanfactor LIN":string caption="Spanfaktor:"
  out "Offset LIN":string caption="Offset:"
  in  "EPA Filename override":T1 caption="eigener Dateiname und Pfad verwenden"
  in  "Conditions:":T59 caption="Prüfbedingung:" items=["field", "laboratory"]
  in  "EPA Filename":T12 caption="File Name"
  in  "EPA Pfad":T9=path "D:/IAG_Data" caption="Pfad"
  in  "EPA PDF erzeugen":T4 caption="SPEICHERN"
  out "Komponentenanzeige EPA":T48 caption="Komponente"
  in  "Gasnummer EPA":T49=1 caption="Komponente:" min=1 max=5
  out "EPA Ausgabetabelle":T60
  out "XY-Graph EPA":cluster{dbl[], dbl[]}[](graph) caption="XY-Graph"
  out "EPA Auswertung":string[][](table) caption="Evaluation"
  in  "Aktiv":T57
  in  "Polynome Speichern":T4 caption="SPEICHERN"
  in  "PolynomAktiv":T57
  in  "PolynomTabelleEingabe":string[][](table)
  out "PolynomTabelleAnzeige":string[][](table)
  in  "Autolin Hovacal":T61=enum."Optionsauswahl 2"
  out "Dynamische Werte":T62 {"Ist Konz 2" format="%#.6f"; "Ist Konz 1" format="%#.6f"; "Ist - Temp" format="%#.1f"; "Wasserkonz." format="%#.4f"; "Drehzahl" format="%#.2f"; "Durchfluss" format="%#.2f"}
  in  "Gase":T63 {"Komponente 2" items=["AIR"]; "Komponente 1" items=["AIR", "O2-20%", "C3H8%2", "NO5000", "MG", "CO2-15%"]; "Trägergas" items=["AIR"]}
  in  "Daten":T64={"Gesamtdurchfluss"=3.0, "Eingangskonzentration \nTrägergas"=0.0, "Eingangskonzentration\nKomponente 1"=0.0, "Eingangskonzentration \nKomponente 2"=0.0, "Ausgangskonzentration \nKomponente 1 "=0.0, "Ausgangskonzentration\nKomponente 2"=0.0, "l/min -> ml/min"=FALSE, "N2 %->ppm"=FALSE, "Komp1 ppm->%"=FALSE, "Komp2ppm->%"=FALSE, "Sollkomp1ppm->%"=FALSE, "Sollkomp2ppm->%"=FALSE} {"Ausgangskonzentration\nKomponente 2" format="%#.4f"; "Eingangskonzentration \nKomponente 2" format="%#.4f"; "Ausgangskonzentration \nKomponente 1" format="%#.4f"; "Eingangskonzentration\nKomponente 1" format="%#.4f"; "Eingangskonzentration \nTrägergas" format="%#.4f"; "Gesamtdurchfluss" format="%#.4f"}
  out "Fehler Kommunikation\nGase":bool
  out "Fehler Kommunikaton\nBetriebsdaten":bool
  out "Fehler Kommunikation\nVaporizer":bool
  in  "Standartwerte Hovacal":bool
  in  "Vaporizer einschalten":bool
  in  "Vaporizer":T65={"Pumpe Ein/Aus"=0.0, "Wasser / Reagent"=0.0, "Reagent dry / wet"=0.0, "Reagent"=4.0, "min. Temperatur\n160 °C"=160.0, "Solltemperatur"=180.0, "Wasserkonzentration\nSoll"=0.0} {"min. Temperatur\n160 °C" min=160.0 format="%#.1f"; "Reagent" items=["HCI", "HF", "NH3", "Hg", "ppm", "Organik"]; "Reagent dry / wet" items=["wet", "dry"]; "Wasser / Reagent" items=["Wasser", "Reagenz"]; "Pumpe Ein/Aus" items=["AUS", "EIN"]}
  out "Komponente HovaCal":T48 caption="Komponente"
  in  "Gasnummer HovaCal":T49=1 caption="Komponente:" min=1 max=5
  in  "SpanTabelleEingabe":string[][](table)
  out "SpanTabelleAnzeige":string[][](table)
  # "Linearisierung"
  # "File Name:"
  # "Pfad:"
  # "zum Deaktivieren kein Beschriftungsfeld \nsondern den Untertitel"
  # "File Name:"
  # "Linearity Check"
  # "Linearitätsnachweis §1065.307"
  # "Aufschaltung Kalibriergas"
  # "Aufschaltpunkt"
  # "Analysator"
  # "Kalibriergas"
  # "Gasteilereinstellungen"
  # "Type:"
  # "Stufen:"
  # "bar"
  # "Kommunikationstreiber:"
  # "Linearisierung allgemein"
  # "IP-Adresse:"
  # "Span Einstellungen"
  # "sec"
  # "%"
  # "sec"
  # "Komponente"
  # "Formel"
  # "Konzentration"
  # "Einheit"
  # "Genauigkeit [%]"
  # "sec"
  # "%"
  # "sec"
  # "Komponente"
  # "Formel"
  # "Konzentration"
  # "Einheit"
  # "Genauigkeit [%]"
  # "sec"
  # "%"
  # "sec"
  # "Komponente"
  # "Formel"
  # "Konzentration"
  # "Einheit"
  # "Genauigkeit [%]"
  # "sec"
  # "%"
  # "sec"
  # "Komponente"
  # "Formel"
  # "Konzentration"
  # "Einheit"
  # "Genauigkeit [%]"
  # "sec"
  # "%"
  # "sec"
  # "Komponente"
  # "Formel"
  # "Konzentration"
  # "Einheit"
  # "Genauigkeit [%]"
  # "sec"
  # "%"
  # "sec"
  # "Komponente"
  # "Formel"
  # "Konzentration"
  # "Einheit"
  # "Genauigkeit [%]"
  # "sec"
  # "%"
  # "sec"
  # "Komponente"
  # "Formel"
  # "Konzentration"
  # "Einheit"
  # "Genauigkeit [%]"
  # "sec"
  # "%"
  # "sec"
  # "Komponente"
  # "Formel"
  # "Konzentration"
  # "Einheit"
  # "Genauigkeit [%]"
  # "sec"
  # "%"
  # "sec"
  # "Komponente"
  # "Formel"
  # "Konzentration"
  # "Einheit"
  # "Genauigkeit [%]"
  # "sec"
  # "%"
  # "sec"
  # "Komponente"
  # "Formel"
  # "Konzentration"
  # "Einheit"
  # "Genauigkeit [%]"
  # "LIN /manuelle Einstellungen"
  # "Pumpe / Syringe-Einstellungen"
  # "MFS Grenzen / Temperatur Einstellungen"
  # "MFC"
  # "Eingang Konzent."
  # "Ausgang Konzent."
  # "Ausgang akt."
  # "Aus. akt. trocken"
  # "Fluss akt"
  # "Fluss Soll"
  # "MFC Konfig"
  # "Komponente fix"
  # "Pumpe"
  # "Pumpe/Spritzen"
  # "Reagenz Sollwert"
  # "Wasser Sollwert %"
  # "Reagenz Aus."
  # "Reag. trocken"
  # "Wasser Aus. %"
  # "W. trocken %"
  # "Drehzahl"
  # "Komponente fix"
  # "Parameter"
  # "Status"
  # "Analysator"
  # "Konstante"
  # "1.Ordnung"
  # "2.Ordnung"
  # "3.Ordnung"
  # "4.Ordnung"
  # "sec."
  # "Konstante"
  # "1.Ordnung"
  # "2.Ordnung"
  # "3.Ordnung"
  # "4.Ordnung"
  # "Pfad:"
  # "File Name:"
  # "Beschreibung der Grenzen:"
  # "Steigung (a1) Wert zwischen 0,99-1,01"
  # "Achsenabschnitt (a0)"
  # "Labor: Wert <=  0,5% von der Kalibriergaskonzentration"
  # "Feld: Wert <=  1% von der Kalibriergaskonzentration"
  # "Bestimmtheitsmaß (R²) Wert >= 0,998"
  # "Standart Fehler (SEE) Wert <= 1% von der Kalibriergaskonzentration"
  # "Linearitätsnachweis §1065.307"
  # "Allgemeine Einstellungen"
  # "Komponenten"
  # "Istwerte"
  # "AutoLIN"
  # "Vaporizer"
